vi "UTF16 Encoding to Unicode (UCS32).vi"(8 "error in":errorcluster, 9 "[UTF-16]":u16[](array[numeric])) -> (0 "error out":errorcluster, 1 "[UCS 32]":u32[](array[numeric]) format="%.0x")   [LabVIEW 2011]
doc: "Decodes the UTF-16 Formatted Unicode numbers."
panel:
  out "UCS 32":u32 format="%.0x"
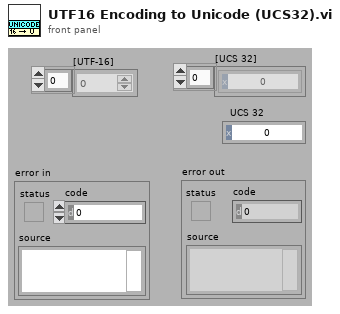
[diagram p1: front panel]
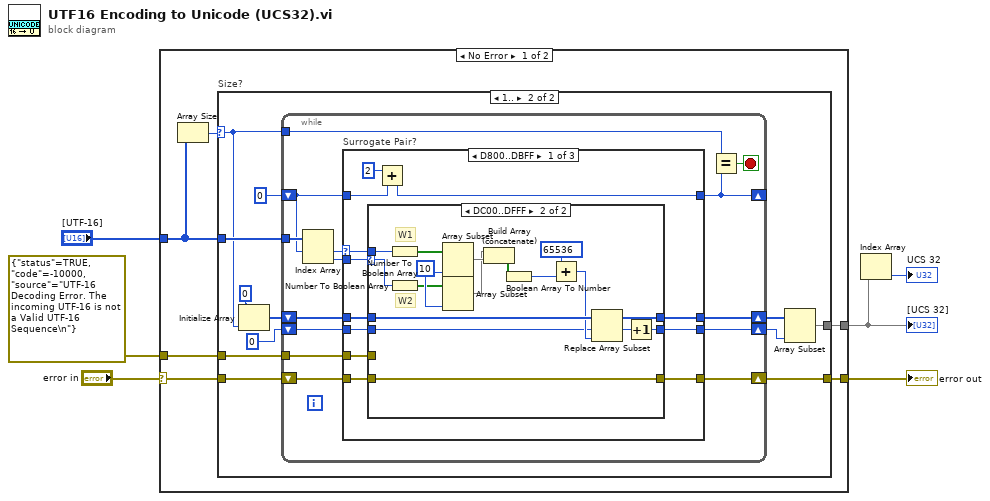
[diagram p0: block diagram]
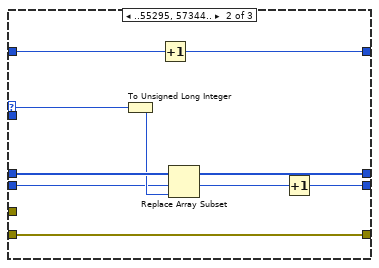
[diagram p4: hidden frame]
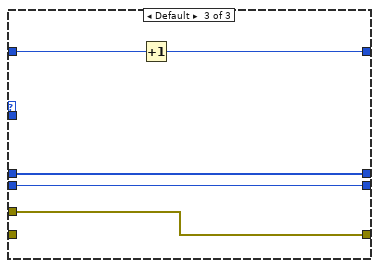
[diagram p5: hidden frame]
diagram:
  n1 = case shown="No Error" "error in" {
    selector: "error in" -> [w10 w85]
    tunnel: "[UTF-16]" -> [w8 _]
    tunnel: [w12 _] -> w1
    tunnel: [w11 w85] -> w4
    tunnel: errorcluster {"status"=TRUE, "code"=-10000, "source"="UTF-16 Decoding Error. The incoming UTF-16 is not a Valid UTF-16 Sequence\n"} ("error IO") -> [w9 _]
    frame No Error {
      n2 = Array Size(array=w8) -> (size(s)=w7:i32)
      n3 = case "Size?" shown="1.." w7 {
        selector: w7 -> [_ w14]
        tunnel: w8 -> [_ w16]
        tunnel: [_ w17] -> w12
        tunnel: [w13 w25] -> w11
        tunnel: w10 -> [w13 w24]
        tunnel: w9 -> [_ w23]
        frame 0, Default {
          # "No input \nNo output"
        }
        frame 1.. {
          n4 = Initialize Array(u32 0 ("UCS"), w14) -> (w21:u32[])
          n5 = while {
            shift-right: [w38] -> w18
            shift-left: w21 -> [w39]
            tunnel: w23 -> [w35]
            shift-right: [w37] -> w25
            shift-left: w24 -> [w36]
            shift-right: [w33] -> w19
            shift-left: 0 -> [w34]
            tunnel: w16 -> [w32]
            shift-right: [w26] -> _
            shift-left: 0 -> [w30]
            tunnel: w14 -> [w27]
            stop <- w29 stop-if-true
            n6 = Index Array(array=w32, index #1=w30) -> (element #1=w31:u16, element #2=w28:u16)  [unwired: 1 in]
            n7 = case "Surrogate Pair?" shown="D800..DBFF" w31 {
              selector: w31 -> [w51 w79 _]
              tunnel: w39 -> [w50 w78 w84]
              tunnel: [w49 w77 w84] -> w38
              tunnel: [w48 w76 w83] -> w37
              tunnel: w36 -> [w47 w76 _]
              tunnel: w35 -> [w46 _ w83]
              tunnel: w34 -> [w45 w74 w82]
              tunnel: [w44 w73 w82] -> w33
              tunnel: w30 -> [w40 w72 w81]
              tunnel: [w42 w71 w80] -> w26
              tunnel: w28 -> [w43 _ _]
              frame 55296..56319 {
                n8 = case shown="DC00..DFFF" w43 {
                  selector: w43 -> [_ w65]
                  tunnel: w51 -> [_ w69]
                  tunnel: w50 -> [w54 w59]
                  tunnel: [w54 w58] -> w49
                  tunnel: [w53 w62] -> w48
                  tunnel: w47 -> [_ w62]
                  tunnel: w46 -> [w53 _]
                  tunnel: w45 -> [w52 w56]
                  tunnel: [w52 w55] -> w44
                  frame Default {
                  }
                  frame 56320..57343 {
                    w70 = 10 ("length")
                    # "W2"
                    # "W1"
                    n9 = Number To Boolean Array(number=w69) -> (Boolean array=w67:bool[])
                    n10 = Number To Boolean Array(number=w65) -> (Boolean array=w66:bool[])
                    n11 = Array Subset(array=w67, length=w70) -> (w61:bool[])  [unwired: 1 in]
                    n12 = Array Subset(array=w66, length=w70) -> (w60:bool[])  [unwired: 1 in]
                    n13 = Build Array (concatenate)(w60, w61) -> (w68:bool[])
                    n14 = Boolean Array To Number(Boolean array=w68) -> (number=w64:u32)
                    n15 = Add(x=u32 65536 ("unsigned 16bit integer"), y=w64) -> (x+y=w57:u32)
                    n16 = Replace Array Subset(array=w59, new element=w57, index=w56) -> (w58:u32[])
                    n17 = Increment(x=w56) -> (x+1=w55:i32)
                  }
                }
                n18 = Add(x=2 ("y"), y=w40) -> (x+y=w42:i32)
              }
              frame ..55295, 57344.. {
                n19 = To Unsigned Long Integer(number=w79) -> (unsigned 32bit integer=w75:u32)
                n20 = Increment(x=w72) -> (x+1=w71:i32)
                n21 = Replace Array Subset(array=w78, new element=w75, index=w74) -> (w77:u32[])
                n22 = Increment(x=w74) -> (x+1=w73:i32)
              }
              frame Default {
                n23 = Increment(x=w81) -> (x+1=w80:i32)
              }
            }
            n24 = Equal?(x=w27, y=w26) -> (x = y?=w29:bool)
          }
          n25 = Array Subset(array=w18, length=w19) -> (w17:u32[])  [unwired: 1 in]
        }
      }
    }
    frame Error {
      # "Do nothing on incoming Error"
    }
  }
  "[UCS 32]" <- w1
  "error out" <- w4
  n26 = Index Array(array=w1) -> (element=→"UCS 32":u32)  [unwired: 1 in]
